vi "UI notifier.vi"(8 "error in (no error)":errorcluster, 10 "Object&State":T1, 11 "Main_Control in":refnum<class "Main_Control.lvclass">) -> (0 "error out":errorcluster, 3 "Main_Control out":refnum<class "Main_Control.lvclass">)   [LabVIEW 2021, in "Main_Control.lvlib" / "Main_Control.lvclass"]
uses:
  Main_Control.lvclass
  notifications.ctl
  Main_Control.lvclass/Main_Control.ctl
  <vilib>/ActorFramework/Message Enqueuer/Message Enqueuer.lvclass/Message Enqueuer.ctl
  <vilib>/ActorFramework/Message Enqueuer/Enqueue.vi
  NI/NI Messages/NI skip one frame AI data Msg/NI skip one frame AI data Msg.lvclass
  C:/Program Files (x86)/National Instruments/LabVIEW 2021/vi.lib/ActorFramework/Message/Message.lvclass
  NI/NI Messages/NI stop task Msg/NI stop task Msg.lvclass
  Camera/Camera Messages/Cam start task Msg/Cam start task Msg.lvclass
  Camera/Camera Messages/Cam stop task Msg/Cam stop task Msg.lvclass
  <vilib>/ActorFramework/Message Priority Queue/Priority Enqueue.vi
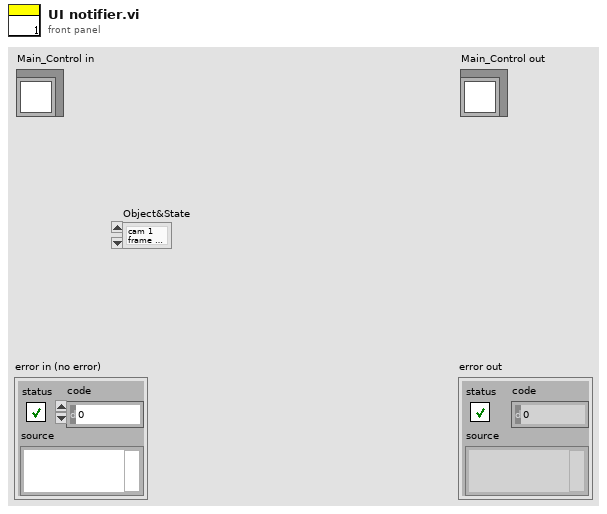
[diagram p1: front panel]
types:
  T1 = typedef "Main_Control.lvlib/Main_Control.lvclass/notifications.ctl" = enum16{"cam 1 frame skkipped", "cam finish", "cam started", "cam stopped", "cam updated", "ni started", "ni stopped", "ni updated"}
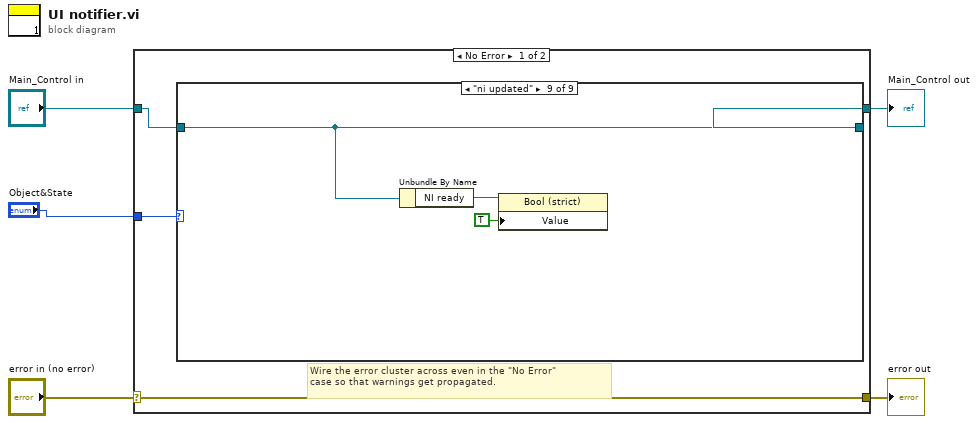
[diagram p0: block diagram]
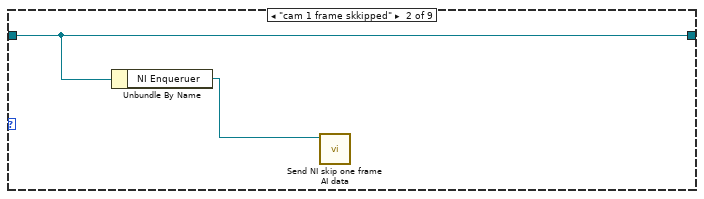
[diagram p3: hidden frame]
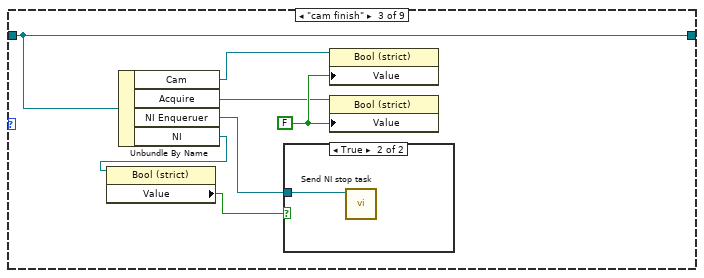
[diagram p4: hidden frame]
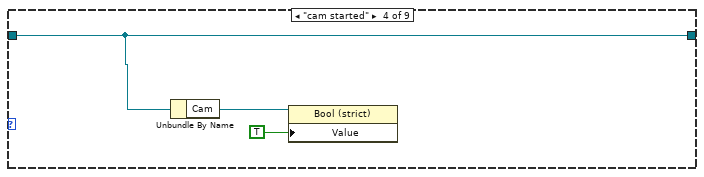
[diagram p6: hidden frame]
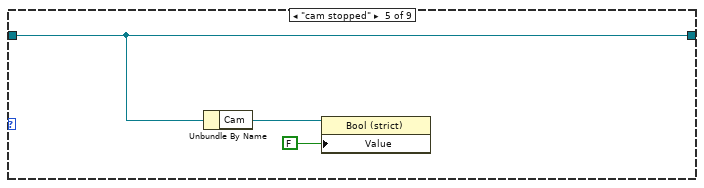
[diagram p7: hidden frame]
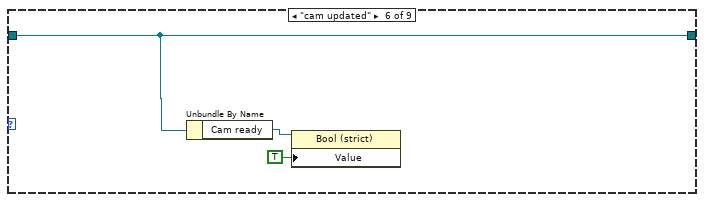
[diagram p8: hidden frame]
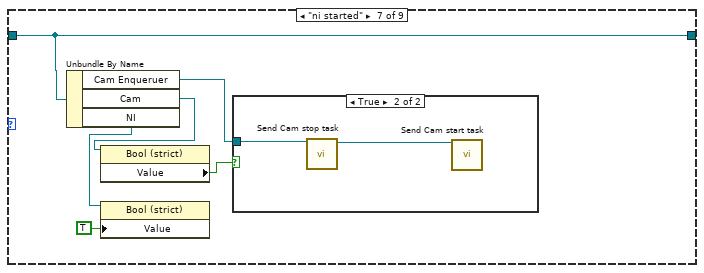
[diagram p9: hidden frame]
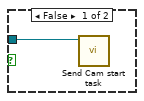
[diagram p10: hidden frame]
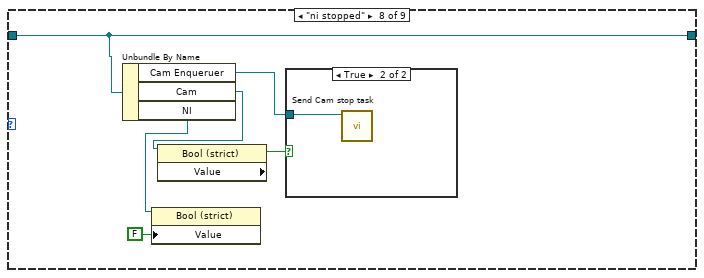
[diagram p11: hidden frame]
diagram:
  n1 = case shown="No Error" "error in (no error)" {
    selector: "error in (no error)" -> [w9 w50]
    tunnel: [w9 w50] -> w4
    tunnel: [w6 w49] -> w2
    tunnel: "Main_Control in" -> [w7 w49]
    tunnel: "Object&State" -> [w8 _]
    frame No Error {
      # "Wire the error cluster across even in the \"No Error\"\ncase so that warnings get propagated."
      n2 = case shown="\"ni updated\"" w8 {
        tunnel: w7 -> [w10 w11 w13 w21 w24 w27 w30 w39 w46]
        tunnel: [w10 w11 w13 w21 w24 w27 w30 w39 w46] -> w6
        frame Default {
        }
        frame "cam 1 frame skkipped" {
          n3 = Unbundle By Name(w11) -> ("NI Enqueruer"=w12:refnum<class "Message Enqueuer.lvclass">)
          n4 = call "Send NI skip one frame AI data.vi"("Message Enqueuer"=w12) -> ()  [unwired: 9 in, 2 out]
        }
        frame "cam finish" {
          w17 = FALSE ("Value")
          n5 = Unbundle By Name(w13) -> ("Cam"=w16:refnum<vi>, "Acquire"=w14:refnum<vi>, "NI Enqueruer"=w15:refnum<class "Message Enqueuer.lvclass">, "NI"=w18:refnum<vi>)
          n6 = property class="Bool (strict)"(reference=w18) -> ("Value"=w19:bool)  [unwired: 1 in, 2 out]
          n7 = case shown="True" w19 {
            tunnel: w15 -> [_ w20]
            frame False {
            }
            frame True {
              n8 = call "Send NI stop task.vi"("Message Enqueuer"=w20) -> ()  [unwired: 9 in, 2 out]
            }
          }
          n9 = property class="Bool (strict)"(reference=w16, "Value"=w17) -> ()  [unwired: 1 in, 2 out]
          n10 = property class="Bool (strict)"(reference=w14, "Value"=w17) -> ()  [unwired: 1 in, 2 out]
        }
        frame "cam started" {
          n11 = Unbundle By Name(w21) -> ("Cam"=w22:refnum<vi>)
          n12 = property class="Bool (strict)"(reference=w22, "Value"=TRUE) -> ()  [unwired: 1 in, 2 out]
        }
        frame "cam stopped" {
          n13 = Unbundle By Name(w24) -> ("Cam"=w25:refnum<vi>)
          n14 = property class="Bool (strict)"(reference=w25, "Value"=FALSE) -> ()  [unwired: 1 in, 2 out]
        }
        frame "cam updated" {
          n15 = Unbundle By Name(w27) -> ("Cam ready"=w29:refnum<vi>)
          n16 = property class="Bool (strict)"(reference=w29, "Value"=TRUE) -> ()  [unwired: 1 in, 2 out]
        }
        frame "ni started" {
          n17 = Unbundle By Name(w30) -> ("Cam Enqueruer"=w31:refnum<class "Message Enqueuer.lvclass">, "Cam"=w32:refnum<vi>, "NI"=w34:refnum<vi>)
          n18 = property class="Bool (strict)"(reference=w32) -> ("Value"=w33:bool)  [unwired: 1 in, 2 out]
          n19 = property class="Bool (strict)"(reference=w34, "Value"=TRUE) -> ()  [unwired: 1 in, 2 out]
          n20 = case shown="True" w33 {
            tunnel: w31 -> [w36 w38]
            frame False {
              n21 = call "Send Cam start task.vi"("Message Enqueuer"=w36) -> ()  [unwired: 9 in, 2 out]
            }
            frame True {
              n22 = call "Send Cam stop task.vi"("Message Enqueuer"=w38) -> ("Message Enqueuer out"=w37:refnum<class "Message Enqueuer.lvclass">)  [unwired: 9 in, 1 out]
              n23 = call "Send Cam start task.vi"("Message Enqueuer"=w37) -> ()  [unwired: 9 in, 2 out]
            }
          }
        }
        frame "ni stopped" {
          n24 = Unbundle By Name(w39) -> ("Cam Enqueruer"=w40:refnum<class "Message Enqueuer.lvclass">, "Cam"=w41:refnum<vi>, "NI"=w44:refnum<vi>)
          n25 = property class="Bool (strict)"(reference=w44, "Value"=FALSE) -> ()  [unwired: 1 in, 2 out]
          n26 = property class="Bool (strict)"(reference=w41) -> ("Value"=w42:bool)  [unwired: 1 in, 2 out]
          n27 = case shown="True" w42 {
            tunnel: w40 -> [_ w45]
            frame False {
            }
            frame True {
              n28 = call "Send Cam stop task.vi"("Message Enqueuer"=w45) -> ()  [unwired: 9 in, 2 out]
            }
          }
        }
        frame "ni updated" {
          n29 = Unbundle By Name(w46) -> ("NI ready"=w47:refnum<vi>)
          n30 = property class="Bool (strict)"(reference=w47, "Value"=TRUE) -> ()  [unwired: 1 in, 2 out]
        }
      }
    }
    frame Error {
    }
  }
  "error out" <- w4
  "Main_Control out" <- w2
